vi "Vision Processing.vi"(4 "error in (no error)":errorcluster, 6 "CameraDevRef":T1) -> ()   [LabVIEW 2011]
uses:
  <vilib>/Rock Robotics/WPI/Camera/WPI_CameraDevRef.ctl
  Robot Global Data.vi
  <vilib>/vision/NI_Vision_Development_Module.lvlib
panel:
  in  "Run Calculations":bool
  out "Raw Turret":dbl
  out "Target X Coord":dbl
  out "Target Distance":dbl
  out "Target Y Coord":dbl
  out "Distance Array":dbl[](array[numeric])
  in  "Scaler":dbl=0.85
  in  "Lower Speed Limit":dbl=0.05
  out "Number of Rectangles Visible":dbl
  out "Y Position Array":dbl[](array[numeric])
  out "X Position Array":dbl[](array[numeric])
  in  "View":bool
  out "Target Info":T2(array[cluster])
  in  "Area Size Limit":i32=444
  in  "Particle Count Limit":i32=8
  in  "Score Limits":T3={"Rect Coverage"=76.0, "Aspect Ratio"=40.0, "X Edge Strength"=40.0, "Y Edge Strength"=60.0}
  in  "Processing":enum32{"Color", "Intensity", "Intensity Open"}(tab)=enum."Intensity Open"
  in  "Luminance":i32=255
  in  "Saturation":i32=255
  in  "Hue":i32(knob)=65 scale=0.0..255.0
  in  "Margins":cluster{"Hue":i32, "Sat":i32, "Lum":i32}={"Hue"=20, "Sat"=27, "Lum"=30} {"Sat" scale=0.0..40.0; "Lum" scale=0.0..40.0; "Hue" scale=0.0..40.0}
  in  "Range":cluster{"Lower value":sgl, "Upper value":sgl}={"Lower value"=150.0, "Upper value"=255.0} {"Lower value" scale=0.0..255.0; "Upper value" scale=0.0..255.0}
  in  "Range":cluster{"Lower value":sgl, "Upper value":sgl}={"Lower value"=123.804344, "Upper value"=255.0} {"Lower value" scale=0.0..255.0; "Upper value" scale=0.0..255.0}
  in  "View":bool
  out "Processed Image":T4(plugin-control)
  out "Original Image":T4(plugin-control)
  # "Instructions:\nProcessing the reflective tape that is illuminated by a ring light can be based\non color or light intensity.\nParticles within the image are scored by rectangle coverage, aspect ratio, and\nfor being hollow with a bold edge. A particle is considered a target if all scores\nare above the score limits. Particles can be annotated -- surrounded by\na rectangle and scores drawn to the left .\nTo control the number of particles being scored, use the count limit and the size\nlimit."
  # "To debug, Enable using the View button.\nFor color processing, you can click in the image to select the color for processing."
  # "Enable by clicking the View button.\nGreen scores are above the limit, orange are below. Inner/outer rect\nindicates all passed."
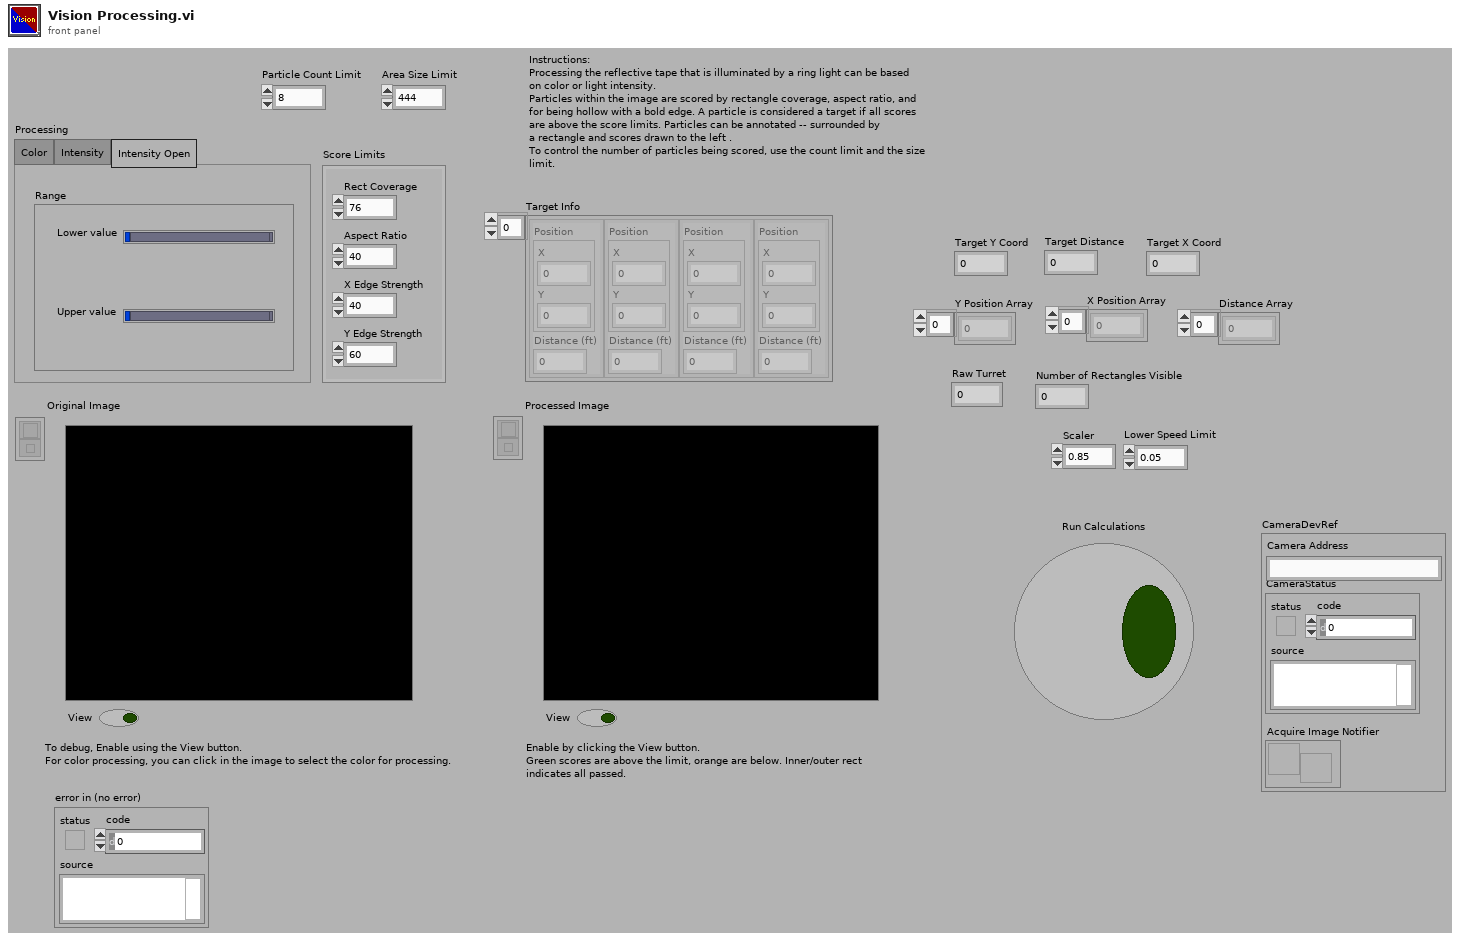
[diagram p1: front panel]
types:
  T1 = typedef "WPI_CameraDevRef.ctl" = cluster{"Camera Address":string, "CameraStatus":errorcluster, "Acquire Image Notifier":refnum<notifier>}
  T2 = cluster{"Position":cluster{"X":dbl, "Y":dbl}, "Distance (ft)":dbl}[]
  T3 = cluster{"Rect Coverage":dbl, "Aspect Ratio":dbl, "X Edge Strength":dbl, "Y Edge Strength":dbl}
  T4 = typedef "IMAQ Image.ctl" = refnum<image>
  T5 = typedef "Image Type" = u32
  T6 = enum32{"AutoM", "Close", "Dilate", "Erode", "Gradient", "Gradient out", "Gradient in", "Hit miss", "Open", "PClose", "POpen", "Thick", "Thin"}
  T7 = typedef "WPI_CameraImageSize.ctl" = enum16{"640x480", "320x240", "160x120"}
  T8 = cluster{"fps":i32, "compression":i32, "Image Size":T7}
  T9 = cluster{cluster{"Left":dbl, "Top":dbl, "Right":dbl, "Bottom":dbl}, dbl[]}[]
  T10 = cluster{"Left":dbl, "Top":dbl, "Right":dbl, "Bottom":dbl}
  T11 = cluster{"Target Center (-1 to 1)":cluster{"X":dbl, "Y":dbl}, "Distance (ft)":dbl}
  T12 = cluster{"Target Center (-1 to 1)":cluster{"X":dbl, "Y":dbl}, "Distance (ft)":dbl}[]
  T13 = typedef "WPI_JoystickDevRef.ctl" = cluster{"Device":T14}
  T14 = typedef "WPI_JoystickDeviceEnum.ctl" = enum16{"USB 1", "USB 2", "USB 3", "USB 4", "Kinect 1", "Kinect 2"}
  T15 = typedef "WPI_JoystickButtonState.ctl" = cluster{"Button 1":bool, "Button 2":bool, "Button 3":bool, "Button 4":bool, "Button 5":bool, "Button 6":bool, "Button 7":bool, "Button 8":bool, "Button 9":bool, "Button 10":bool, "Button 11":bool, "Button 12":bool}
  T16 = cluster{"axis 1 (x)":dbl, "axis 2 (y)":dbl, "axis 3 (throttle)":dbl, "axis 4":dbl, "axis 5":dbl, "axis 6":dbl}
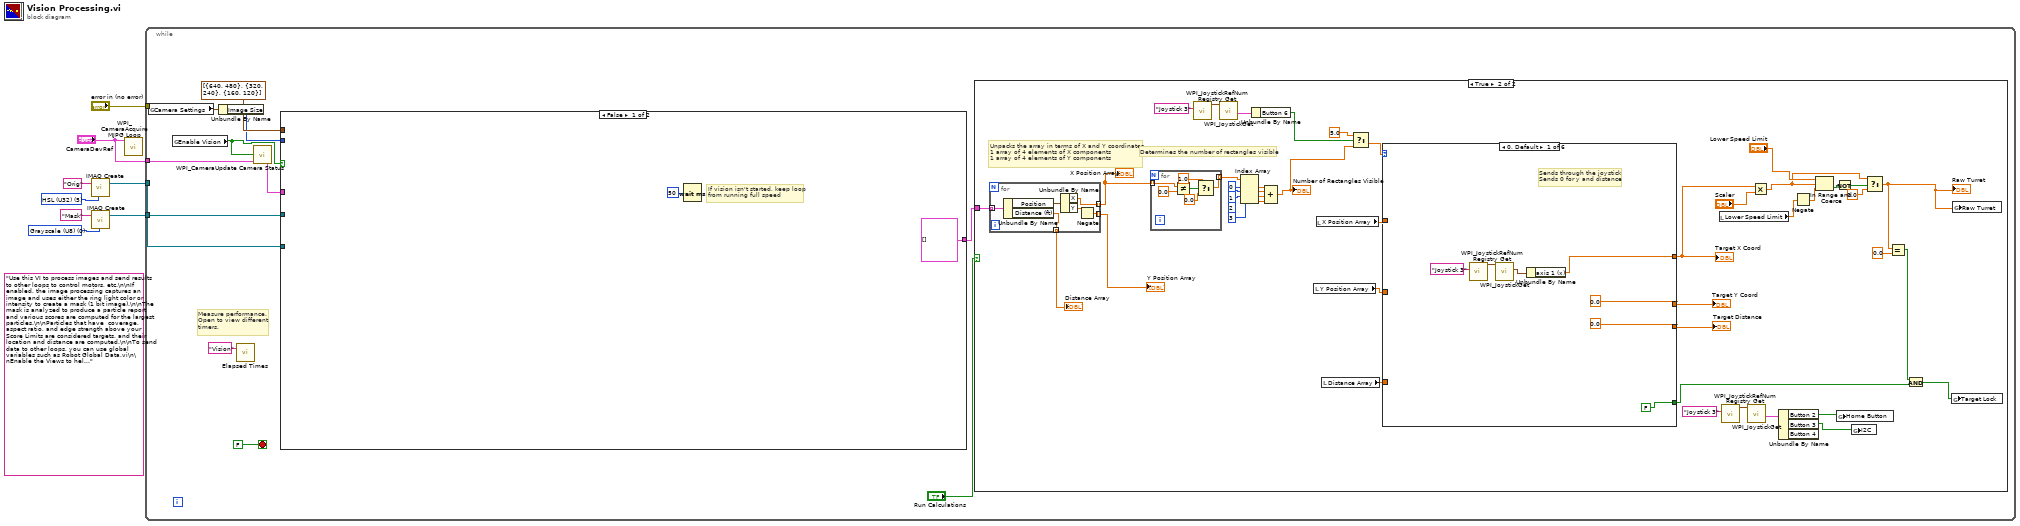
[diagram p0: block diagram]
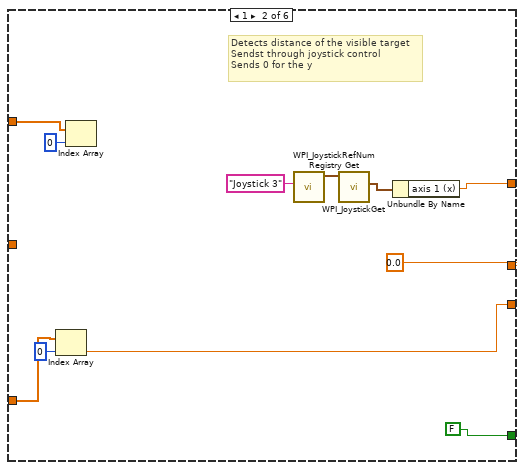
[diagram p3: hidden frame]
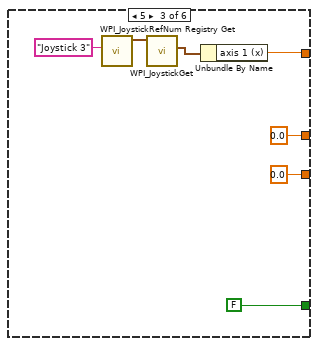
[diagram p4: hidden frame]
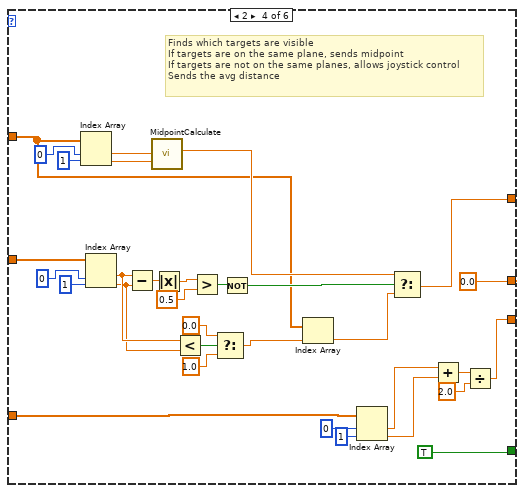
[diagram p5: hidden frame]
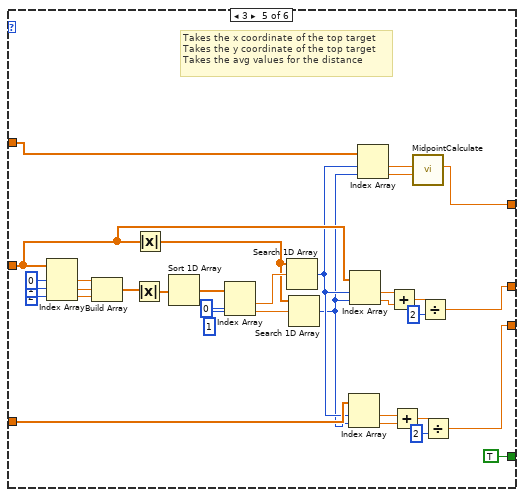
[diagram p6: hidden frame]
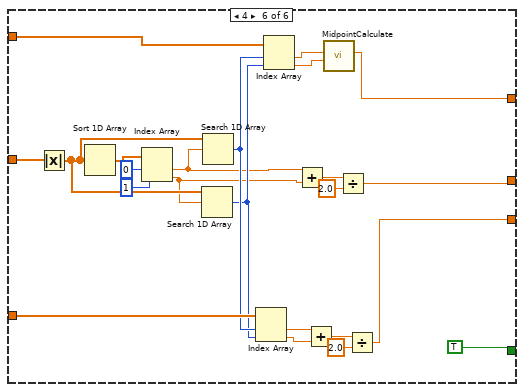
[diagram p7: hidden frame]
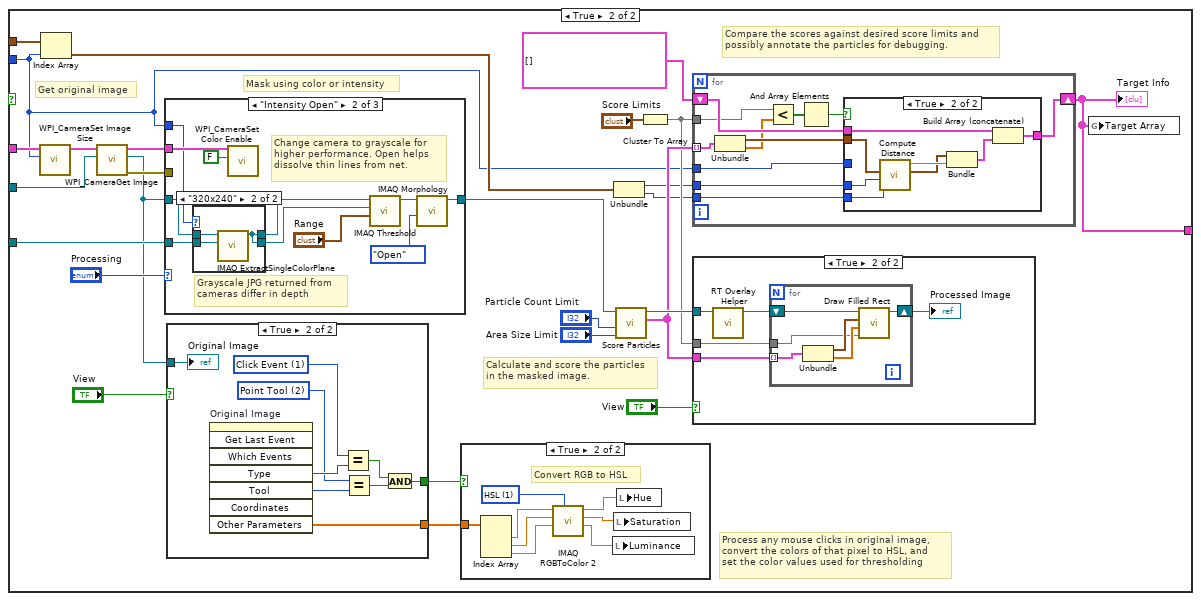
[diagram p8: hidden frame]
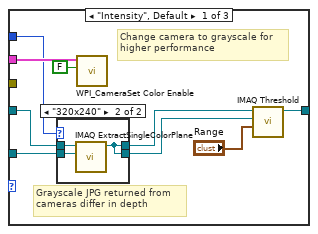
[diagram p10: hidden frame]
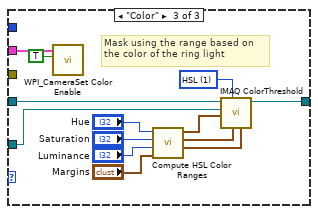
[diagram p13: hidden frame]
diagram:
  w3 = T5 0 items=["Grayscale (U8)", "Grayscale (I16)", "Grayscale (SGL)", "Complex (CSG)", "RGB (U32)", "HSL (U32)", "RGB (U64)", "Grayscale (U16)"] ("Image Type")
  (unwired) "Use this VI to process images and send results to other loops to control motors, etc.\n\nIf enabled, the image processing captures an image and uses either the ring light color or intensity to create a mask (1 bit image).\n\nThe mask is analyzed to produce a particle report and various scores are computed for the largest particles.\n\nParticles that have  coverage, aspect ratio, and edge strength above your Score Limits are considered targets, and their location and distance are computed.\n\nTo send data to other loops, you can use global variables such as Robot Global Data.vi\n\nEnable the Views to help debug color settings. Disable the View to speed up processing."
  w7 = T5 5 items=["Grayscale (U8)", "Grayscale (I16)", "Grayscale (SGL)", "Complex (CSG)", "RGB (U32)", "HSL (U32)", "RGB (U64)", "Grayscale (U16)"] ("Image Type")
  n1 = call "IMAQ Create"("Image Name"="Orig", "Image Type"=w7) -> ("New Image"=w6:T4)  [unwired: 2 in, 2 out]
  n2 = call "IMAQ Create"("Image Name"="Mask", "Image Type"=w3) -> ("New Image"=w1:T4)  [unwired: 2 in, 2 out]
  n3 = call <vilib>:"WPI_CameraAcquire MJPG Loop.vi"("CameraDevRef"="CameraDevRef") -> ()  [unwired: 11 in]
  n4 = while {
    tunnel: w6 -> [w19]
    tunnel: "CameraDevRef" -> [w18]
    tunnel: "error in (no error)" -> [_]
    tunnel: w1 -> [w14]
    stop <- FALSE stop-if-true
    # "Measure performance.\nOpen to view different\ntimers."
    n5 = global read "Robot Global Data.vi" "Camera Settings"() -> (w12:T8)
    n6 = global read "Robot Global Data.vi" "Enable Vision"() -> (w16:bool)
    n7 = Unbundle By Name(w12) -> ("Image Size"=w11:T7)
    n8 = call "Elapsed Times.vi"("Call Name"="Vision") -> ()  [unwired: 2 in, 1 out]
    n9 = call <vilib>:"WPI_CameraUpdate Camera Status.vi"("CameraDevRef In"=w18, "Enable Vision"=w16) -> ("CameraDevRef Out"=w17:T1)  [unwired: 3 in]
    n10 = case shown="False" w16 {
      tunnel: w19 -> [_ w208]
      tunnel: w17 -> [_ w204]
      tunnel: w14 -> [_ w195]
      tunnel: cluster{i32, i32}[] [{640, 480}, {320, 240}, {160, 120}] -> [_ w199]
      tunnel: w11 -> [_ w192]
      tunnel: [T2 [] w193] -> w10
      frame False {
        # "If vision isn't started, keep loop\nfrom running full speed"
        n11 = Wait (ms)(milliseconds to wait=u32 50) -> ()  [unwired: 1 out]
      }
      frame True {
        # "Compare the scores against desired score limits and\npossibly annotate the particles for debugging."
        # "Process any mouse clicks in original image,\nconvert the colors of that pixel to HSL, and\nset the color values used for thresholding"
        # "Calculate and score the particles\nin the masked image."
        # "Mask using color or intensity"
        # "Get original image"
        n12 = call <vilib>:"WPI_CameraSet Image Size.vi"("Image Size"=w192, "CameraDevRef"=w204) -> ("CameraDevRef Out"=w205:T1)  [unwired: 8 in, 1 out]
        n13 = Index Array(array=w199, index=w192) -> (element=w196:cluster{i32, i32})
        n14 = call <vilib>:"WPI_CameraGet Image.vi"("Image"=w208, "CameraDevRef"=w205) -> ("error out"=w206:errorcluster, "Image Out"=w194:T4, "CameraDevRef Out"=w207:T1)  [unwired: 7 in]
        n15 = case shown="\"Intensity Open\"" "Processing" {
          tunnel: w194 -> [w230 w242 w268]
          tunnel: [w233 w247 w267] -> w202
          tunnel: w207 -> [w231 w245 w258]
          tunnel: w206 -> [_ _ _]
          tunnel: w195 -> [w229 w243 w256]
          tunnel: w192 -> [w228 w244 _]
          frame "Intensity", Default {
            # "Grayscale JPG returned from\ncameras differ in depth"
            # "Change camera to grayscale for\nhigher performance"
            n16 = case shown="\"320x240\"" w228 {
              tunnel: w230 -> [w236 w239]
              tunnel: w229 -> [w235 w238]
              tunnel: [w236 w237] -> w227
              tunnel: [w235 w237] -> w226
              frame "640x480", Default {
              }
              frame "320x240" {
                n17 = call "IMAQ ExtractSingleColorPlane"("Image Dst"=w238, "Image Src"=w239) -> ("Image Dst Out"=w237:T4)  [unwired: 8 in, 1 out]
              }
            }
            n18 = call <vilib>:"WPI_CameraSet Color Enable.vi"("Color Enabled"=FALSE, "CameraDevRef"=w231) -> ()  [unwired: 8 in, 2 out]
            n19 = call "IMAQ Threshold"("Range"="Range", "Image Dst"=w226, "Image Src"=w227) -> ("Image Dst Out"=w233:T4)  [unwired: 3 in, 5 out]
          }
          frame "Intensity Open" {
            # "Grayscale JPG returned from\ncameras differ in depth"
            # "Change camera to grayscale for\nhigher performance. Open helps\ndissolve thin lines from net."
            n20 = case shown="\"320x240\"" w244 {
              tunnel: w242 -> [w252 w255]
              tunnel: w243 -> [w251 w254]
              tunnel: [w252 w253] -> w241
              tunnel: [w251 w253] -> w240
              frame "640x480", Default {
              }
              frame "320x240" {
                n21 = call "IMAQ ExtractSingleColorPlane"("Image Dst"=w254, "Image Src"=w255) -> ("Image Dst Out"=w253:T4)  [unwired: 8 in, 1 out]
              }
            }
            n22 = call <vilib>:"WPI_CameraSet Color Enable.vi"("Color Enabled"=FALSE, "CameraDevRef"=w245) -> ()  [unwired: 8 in, 2 out]
            n23 = call "IMAQ Threshold"("Range"="Range", "Image Dst"=w240, "Image Src"=w241) -> ("Image Dst Out"=w248:T4)  [unwired: 3 in, 5 out]
            n24 = call "IMAQ Morphology"("Operation"=T6."Open", "Image Src"=w248) -> ("Image Dst Out"=w247:T4)  [unwired: 8 in, 1 out]
          }
          frame "Color" {
            w266 = u16 1 items=["RGB", "HSL", "HSV", "HSI"] ("Color Mode")
            # "Mask using the range based on\nthe color of the ring light"
            n25 = call <vilib>:"WPI_CameraSet Color Enable.vi"("Color Enabled"=TRUE, "CameraDevRef"=w258) -> ()  [unwired: 8 in, 2 out]
            n26 = call "Compute HSL Color Ranges.vi"("Margins"="Margins", "Luminance"="Luminance", "Saturation"="Saturation", "Hue"="Hue") -> ("Lum Range"=w263:cluster{i32, i32}, "Sat Range"=w264:cluster{i32, i32}, "Hue Range"=w265:cluster{i32, i32})  [unwired: 5 in]
            n27 = call "IMAQ ColorThreshold"("Blue or Luma or Val or Inten Range"=w263, "Green or Sat Range"=w264, "Color Mode"=w266, "Red or Hue Range"=w265, "Image Dst"=w256, "Image Src"=w268) -> ("Image Dst Out"=w267:T4)  [unwired: 4 in, 1 out]
          }
        }
        n28 = case shown="True" "View" {
          tunnel: w194 -> [_ w288]
          tunnel: [_ w283] -> w201
          tunnel: [_ w280] -> w200
          frame False {
          }
          frame True {
            w281 = 2 items=["None", "Selection Tool", "Point Tool", "Line Tool", "Rectangle Tool", "Oval Tool", "Polygon Tool", "ClosedFreehandTool", "Annulus Tool", "Rotated Rectangle Tool", "Zoom Tool", "Pan Tool", "Polyline Tool", "Freehand Tool"] ("Tool")
            w282 = 1 items=["No Event"=0, "Click Event"=1, "Draw Event"=2, "Size Event"=4, "Scroll Event"=5, "Double Click Event"=8] ("Type")
            n29 = invoke on="Original Image" class="ImageControl" method="Get Last Event"() -> ("Type"=w284:i32, "Tool"=w287:i32, "Other Parameters"=w280:sgl[])  [unwired: 8 in, 5 out]
            n30 = Equal?(x=w282, y=w284) -> (x = y?=w285:bool)
            n31 = Equal?(x=w281, y=w287) -> (x = y?=w286:bool)
            n32 = And(x=w285, y=w286) -> (x .and. y?=w283:bool)
            "Original Image" <- w288
          }
        }
        n33 = case shown="True" w201 {
          tunnel: w200 -> [_ w225]
          frame False {
          }
          frame True {
            w224 = u16 1 items=["RGB", "HSL", "HSV", "HSI", "CIE L*a*b*", "CIE XYZ"] ("Color Mode")
            # "Convert RGB to HSL"
            n34 = Index Array(array=w225) -> (element #1=w223:sgl, element #2=w221:sgl, element #3=w219:sgl)  [unwired: 3 in]
            n35 = call "IMAQ RGBToColor 2"("Color Mode"=w224, "Blue value"=w219, "Green value"=w221, "Red value"=w223) -> ("Blue or Luma or Val or Inten or Z or b*value"=w218:dbl, "Green or Sat or Y or a* value"=w220:dbl, "Red or Hue or X or L* value"=w222:dbl)  [unwired: 4 in, 1 out]
            n36 = local write "Luminance"(w218) -> ()
            n37 = local write "Saturation"(w220) -> ()
            n38 = local write "Hue"(w222) -> ()
          }
        }
        n39 = Unbundle(w196) -> (w198:i32, w197:i32)
        n40 = call "Score Particles.vi"("Area Size Limit"="Area Size Limit", "Particle Count Limit"="Particle Count Limit", "Image Refnum in"=w202) -> ("Scored Particle Info"=w213:T9, "Image Refnum out"=w216:T4)  [unwired: 7 in]
        n41 = Cluster To Array(cluster="Score Limits") -> (array=w211:dbl[])
        n42 = for {
          shift-right: [w298] -> w193
          shift-left: T2 [] -> [w299]
          tunnel: w198 -> [w297]
          tunnel: w213 -> [w295] mode=indexing
          tunnel: w211 -> [w290]
          tunnel: w192 -> [w294]
          tunnel: w197 -> [w289]
          n43 = Unbundle(w295) -> (w296:T10, w291:dbl[])
          n44 = Less?(x=w290, y=w291) -> (x < y?=w293:bool[])
          n45 = And Array Elements(Boolean array=w293) -> (logical AND=w292:bool)
          n46 = case shown="True" w292 {
            tunnel: w299 -> [w300 w308]
            tunnel: [w300 w307] -> w298
            tunnel: w296 -> [_ w303]
            tunnel: w297 -> [_ w305]
            tunnel: w294 -> [_ _]
            tunnel: w289 -> [_ w302]
            frame False {
            }
            frame True {
              n47 = call "Compute Distance.vi"("Y Image Resolution"=w302, "X Image Resolution"=w305, "Bounding Box"=w303) -> ("Target Center (-1 to 1)"=w301:cluster{"X":dbl, "Y":dbl}, "Distance (ft)"=w304:dbl)  [unwired: 7 in]
              n48 = Bundle("Target Center (-1 to 1)"=w301, "Distance (ft)"=w304) -> (w306:T11)  [unwired: 1 in]
              n49 = Build Array (concatenate)(w308, w306) -> (w307:T12)
            }
          }
        }
        "Target Info" <- w193
        n50 = case shown="True" "View" {
          tunnel: w216 -> [_ w270]
          tunnel: w213 -> [_ w272]
          tunnel: w211 -> [_ w271]
          frame False {
          }
          frame True {
            n51 = call "RT Overlay Helper.vi"("Refnum in"=w270) -> ("Refnum out"=w273:T4)  [unwired: 10 in]
            n52 = for {
              shift-right: [w278] -> w269
              shift-left: w273 -> [w279]
              tunnel: w272 -> [w275] mode=indexing
              tunnel: w271 -> [w274]
              n53 = Unbundle(w275) -> (w276:T10, w277:dbl[])
              n54 = call "Draw Filled Rect.vi"("Limits"=w274, "Scores"=w277, "Bounding Box"=w276, "image in"=w279) -> ("image out"=w278:T4)  [unwired: 7 in]
            }
            "Processed Image" <- w269
          }
        }
        n55 = global write "Robot Global Data.vi" "Target Array"(w193) -> ()
      }
    }
    n56 = case shown="True" "Run Calculations" {
      tunnel: w10 -> [_ w36]
      frame False {
      }
      frame True {
        # "Determines the number of rectangles visible"
        # "Unpacks the array in terms of X and Y coordinates\n1 array of 4 elements of X components\n1 array of 4 elements of Y components"
        n57 = for {
          tunnel: [w187] -> w37 mode=indexing
          tunnel: [w188] -> w47 mode=indexing
          tunnel: w36 -> [w185] mode=indexing
          tunnel: [w184] -> w56 mode=indexing
          n58 = Unbundle By Name(w185) -> ("Position"=w189:cluster{"X":dbl, "Y":dbl}, "Distance (ft)"=w184:dbl)
          n59 = Unbundle By Name(w189) -> ("X"=w188:dbl, "Y"=w186:dbl)
          n60 = Negate(x=w186) -> (-x=w187:dbl)
        }
        "X Position Array" <- w47
        "Y Position Array" <- w37
        "Distance Array" <- w56
        n61 = for {
          tunnel: w47 -> [w69] mode=indexing
          tunnel: [w65] -> w46 mode=indexing
          n62 = Not Equal?(x=w69, y=0.0) -> (x != y?=w68:bool)
          n63 = Select(t=1.0, s=w68, f=0.0) -> (s? t:f=w65:dbl)
        }
        n64 = call <vilib>:"WPI_JoystickRefNum Registry Get.vi"("refnum name"="Joystick 3") -> ("JoystickDevRef"=w25:T13)  [unwired: 9 in, 1 out]
        n65 = call <vilib>:"WPI_JoystickGet.vi"("JoystickDevRef"=w25) -> ("Buttons"=w23:T15)  [unwired: 4 in, 2 out]
        n66 = Index Array(array=w46, index #1=0 ("index"), index #2=1 ("index"), index #3=2 ("index"), index #4=3 ("index")) -> (element #1=w44:dbl, element #2=w45:dbl, element #3=w43:dbl, element #4=w42:dbl)
        n67 = Unbundle By Name(w23) -> ("Button 6"=w22:bool)
        n68 = Compound Arithmetic op=ADD(w44, w45, w43, w42) -> (w35:dbl)
        "Number of Rectangles Visible" <- w35
        n69 = local read "Y Position Array"() -> (w60:dbl[])
        n70 = local read "X Position Array"() -> (w48:dbl[])
        n71 = local read "Distance Array"() -> (w61:dbl[])
        n72 = Select(t=5.0, s=w22, f=w35) -> (s? t:f=w63:dbl)
        n73 = case shown="0, Default" w63 {
          tunnel: w48 -> [_ w83 _ w98 w144 w177]
          tunnel: [w71 w78 w89 w116 w141 w167] -> w59
          tunnel: [0.0 ("X") 0.0 ("X") 0.0 ("X") 0.0 ("X") w145 w166] -> w57
          tunnel: [0.0 ("X") w86 0.0 ("X") w109 w129 w161] -> w58
          tunnel: w60 -> [_ _ _ w125 w137 w182]
          tunnel: w61 -> [_ w88 _ w108 w132 w176]
          tunnel: [FALSE FALSE FALSE TRUE TRUE TRUE] -> w32
          frame 0, Default {
            # "Sends through the joystick\nSends 0 for y and distance"
            n74 = call <vilib>:"WPI_JoystickRefNum Registry Get.vi"("refnum name"="Joystick 3") -> ("JoystickDevRef"=w74:T13)  [unwired: 9 in, 1 out]
            n75 = call <vilib>:"WPI_JoystickGet.vi"("JoystickDevRef"=w74) -> ("Axes"=w72:T16)  [unwired: 4 in, 2 out]
            n76 = Unbundle By Name(w72) -> ("axis 1 (x)"=w71:dbl)
          }
          frame 1 {
            # "Detects distance of the visible target\nSendst through joystick control\nSends 0 for the y"
            n77 = Index Array(array=w88, index=0) -> (element=w86:dbl)
            n78 = Index Array(array=w83, index=0) -> ()  [unwired: 1 out]
            n79 = call <vilib>:"WPI_JoystickRefNum Registry Get.vi"("refnum name"="Joystick 3") -> ("JoystickDevRef"=w81:T13)  [unwired: 9 in, 1 out]
            n80 = call <vilib>:"WPI_JoystickGet.vi"("JoystickDevRef"=w81) -> ("Axes"=w79:T16)  [unwired: 4 in, 2 out]
            n81 = Unbundle By Name(w79) -> ("axis 1 (x)"=w78:dbl)
          }
          frame 5 {
            n82 = call <vilib>:"WPI_JoystickRefNum Registry Get.vi"("refnum name"="Joystick 3") -> ("JoystickDevRef"=w92:T13)  [unwired: 9 in, 1 out]
            n83 = call <vilib>:"WPI_JoystickGet.vi"("JoystickDevRef"=w92) -> ("Axes"=w90:T16)  [unwired: 4 in, 2 out]
            n84 = Unbundle By Name(w90) -> ("axis 1 (x)"=w89:dbl)
          }
          frame 2 {
            # "Finds which targets are visible\nIf targets are on the same plane, sends midpoint\nIf targets are not on the same planes, allows joystick control\nSends the avg distance"
            n85 = Index Array(array=w98, index #1=0 ("index"), index #2=1 ("index")) -> (element #1=w114:dbl, element #2=w113:dbl)
            n86 = Index Array(array=w125, index #1=0 ("index"), index #2=1 ("index")) -> (element #1=w104:dbl, element #2=w103:dbl)
            n87 = Subtract(x=w104, y=w103) -> (x-y=w122:dbl)
            n88 = call "MidpointCalculate.vi"("X2"=w113, "X1"=w114) -> ("Midpoint"=w117:dbl)  [unwired: 9 in]
            n89 = Absolute Value(x=w122) -> (abs(x)=w121:dbl)
            n90 = Less?(x=w104, y=w103) -> (x < y?=w102:bool)
            n91 = Greater?(x=w121, y=0.5) -> (0:w118:bool)
            n92 = Select(t=0.0, s=w102, f=1.0) -> (s? t:f=w99:dbl)
            n93 = Not(x=w118) -> (.not. x?=w119:bool)
            n94 = Index Array(array=w98, index=w99) -> (element=w97:dbl)
            n95 = Index Array(array=w108, index #1=0 ("index"), index #2=1 ("index")) -> (element #1=w107:dbl, element #2=w106:dbl)
            n96 = Select(t=w117, s=w119, f=w97) -> (s? t:f=w116:dbl)
            n97 = Add(x=w107, y=w106) -> (x+y=w112:dbl)
            n98 = Divide(x=w112, y=2.0) -> (x/y=w109:dbl)
          }
          frame 3 {
            # "Takes the x coordinate of the top target\nTakes the y coordinate of the top target\nTakes the avg values for the distance"
            n99 = Index Array(array=w137, index #1=0 ("index"), index #2=1 ("index"), index #3=2 ("index")) -> (element #1=w157:dbl, element #2=w156:dbl, element #3=w155:dbl)
            n100 = Build Array(w157, w156, w155) -> (w154:dbl[])
            n101 = Absolute Value(x=w154) -> (abs(x)=w148:dbl[])
            n102 = Absolute Value(x=w137) -> (abs(x)=w140:dbl[])
            n103 = Sort 1D Array(array=w148) -> (sorted array=w153:dbl[])
            n104 = Index Array(array=w153, index #1=0 ("index"), index #2=1 ("index")) -> (element #1=w149:dbl, element #2=w150:dbl)
            n105 = Search 1D Array(1D array=w140, element=w149) -> (index of element=w131:i32)  [unwired: 1 in]
            n106 = Search 1D Array(1D array=w140, element=w150) -> (index of element=w130:i32)  [unwired: 1 in]
            n107 = Index Array(array=w132, index #1=w131, index #2=w130) -> (element #1=w134:dbl, element #2=w133:dbl)
            n108 = Index Array(array=w137, index #1=w131, index #2=w130) -> (element #1=w139:dbl, element #2=w138:dbl)
            n109 = Index Array(array=w144, index #1=w131, index #2=w130) -> (element #1=w143:dbl, element #2=w142:dbl)
            n110 = Add(x=w139, y=w138) -> (x+y=w147:dbl)
            n111 = Add(x=w134, y=w133) -> (x+y=w135:dbl)
            n112 = call "MidpointCalculate.vi"("X2"=w142, "X1"=w143) -> ("Midpoint"=w141:dbl)  [unwired: 9 in]
            n113 = Divide(x=w147, y=2) -> (x/y=w145:dbl)
            n114 = Divide(x=w135, y=2) -> (x/y=w129:dbl)
          }
          frame 4 {
            n115 = Absolute Value(x=w182) -> (abs(x)=w178:dbl[])
            n116 = Sort 1D Array(array=w178) -> (sorted array=w181:dbl[])
            n117 = Index Array(array=w181, index #1=0 ("index"), index #2=1 ("index")) -> (element #1=w173:dbl, element #2=w172:dbl)
            n118 = Search 1D Array(1D array=w178, element=w172) -> (index of element=w174:i32)  [unwired: 1 in]
            n119 = Search 1D Array(1D array=w178, element=w173) -> (index of element=w175:i32)  [unwired: 1 in]
            n120 = Index Array(array=w176, index #1=w175, index #2=w174) -> (element #1=w163:dbl, element #2=w162:dbl)
            n121 = Index Array(array=w177, index #1=w175, index #2=w174) -> (element #1=w169:dbl, element #2=w168:dbl)
            n122 = Add(x=w173, y=w172) -> (x+y=w171:dbl)
            n123 = Add(x=w163, y=w162) -> (x+y=w164:dbl)
            n124 = call "MidpointCalculate.vi"("X2"=w168, "X1"=w169) -> ("Midpoint"=w167:dbl)  [unwired: 9 in]
            n125 = Divide(x=w171, y=2.0) -> (x/y=w166:dbl)
            n126 = Divide(x=w164, y=2.0) -> (x/y=w161:dbl)
          }
        }
        "Target Y Coord" <- w57
        "Target Distance" <- w58
        "Target X Coord" <- w59
        n127 = local read "Lower Speed Limit"() -> (w50:dbl)
        n128 = call <vilib>:"WPI_JoystickRefNum Registry Get.vi"("refnum name"="Joystick 3") -> ("JoystickDevRef"=w29:T13)  [unwired: 9 in, 1 out]
        n129 = call <vilib>:"WPI_JoystickGet.vi"("JoystickDevRef"=w29) -> ("Buttons"=w27:T15)  [unwired: 4 in, 2 out]
        n130 = Multiply(x=w59, y="Scaler") -> (x*y=w55:dbl)
        n131 = Unbundle By Name(w27) -> ("Button 2"=w26:bool, "Button 3"=w21:bool)  [unwired: 1 out]
        n132 = Negate(x=w50) -> (-x=w51:dbl)
        n133 = In Range and Coerce(upper limit="Lower Speed Limit", x=w55, lower limit=w51) -> (In Range?=w52:bool)  [unwired: 1 out]
        n134 = Not(x=w52) -> (.not. x?=w53:bool)
        n135 = global write "Robot Global Data.vi" "Home Button"(w26) -> ()
        n136 = global write "Robot Global Data.vi" "I2C"(w21) -> ()
        n137 = Select(t=w55, s=w53, f=0.0) -> (s? t:f=w34:dbl)
        "Raw Turret" <- w34
        n138 = Equal?(x=w34, y=0.0) -> (x = y?=w31:bool)
        n139 = And(x=w31, y=w32) -> (x .and. y?=w30:bool)
        n140 = global write "Robot Global Data.vi" "Target Lock"(w30) -> ()
        n141 = global write "Robot Global Data.vi" "Raw Turret"(w34) -> ()
      }
    }
  }
